vi "JiaxinInitDone.vi"(8 "error in (no error)":errorcluster, 10 "InstrumentData":T1, 11 "TranslationStageUI.lvclass":refnum<class "TranslationStageUI.lvclass">) -> (0 "error out":errorcluster, 3 "TranslationStageUI.lvclass":refnum<class "TranslationStageUI.lvclass">)   [LabVIEW 2023, in "TranslationStage_UI.lvlib" / "TranslationStageUI.lvclass"]
uses:
  TranslationStageUI.lvclass
  typedefs/InstrumentData.ctl
  typedefs/instrumentType.ctl
  TranslationStageUI.lvclass/TranslationStageUI.ctl
  typedefs/typedefs.lvlib
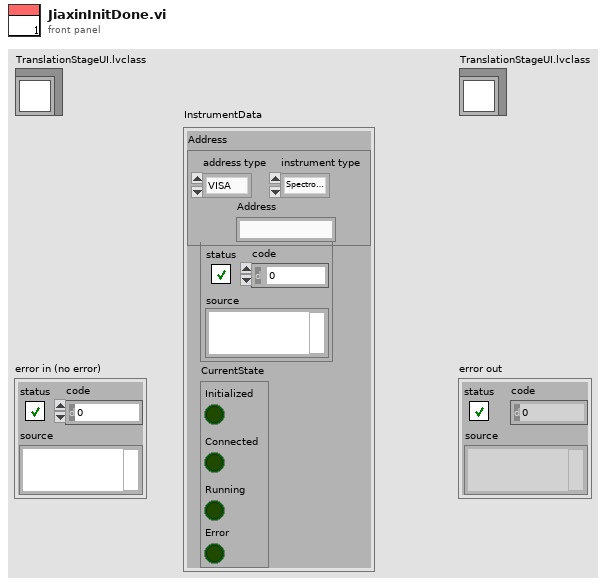
[diagram p1: front panel]
types:
  T1 = typedef "typedefs.lvlib/InstrumentData.ctl" = cluster{"Instr Error":errorcluster, "Address":cluster{"address type":enum16{"VISA", "Index"}, "Address":string, "instrument type":T2}, "CurrentState":cluster{"Initialized":bool, "Connected":bool, "Running":bool, "Error":bool}}
  T2 = typedef "typedefs.lvlib/instrumentType.ctl" = enum16{"Spectrometer", "Camera", "Stepper", "Piezo"}
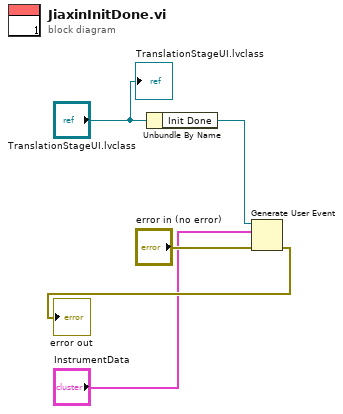
[diagram p0: block diagram]
diagram:
  n1 = Unbundle By Name("TranslationStageUI.lvclass") -> ("Init Done"=w5:refnum<user-event>)
  n2 = Generate User Event(user event=w5, event data cluster="InstrumentData", error in="error in (no error)") -> (error out=→"error out":errorcluster)  [unwired: 1 in, 1 out]
  "TranslationStageUI.lvclass" <- "TranslationStageUI.lvclass"
